vi "Load data.vi"(0 "File style in":u16(ring) items=["Sequential files", "Single database"], 1 "Fixed style":bool, 5 "Xcol in":i16, 7 "Ycol in":i16, 9 "Files in":path[](array[path]), 11 "Delim in":string) -> (4 "File style out":u16(ring) items=["Sequential files", "Single database"], 6 "Xcol out":i16, 8 "Ycol out":i16, 10 "Files out":path[](array[path]), 15 "Delim out":string)   [LabVIEW 2014]
panel:
  out "Delim":string
  in  "Ycol":i16=1
  in  "Xcol":i16
  out "Files":path[](array[path])
  in  "Process Stop Button":bool
  in  "File style":u16(ring) items=["Sequential files", "Single database"]
  in  "File delimit":u16(ring) items=["Tab", "Comma"]
  in  "Open Button":bool
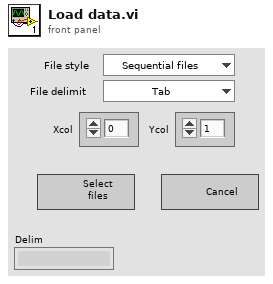
[diagram p1: front panel]
types:
  T1 = enum8{"Enabled", "Disabled", "Disabled and Grayed Out"}
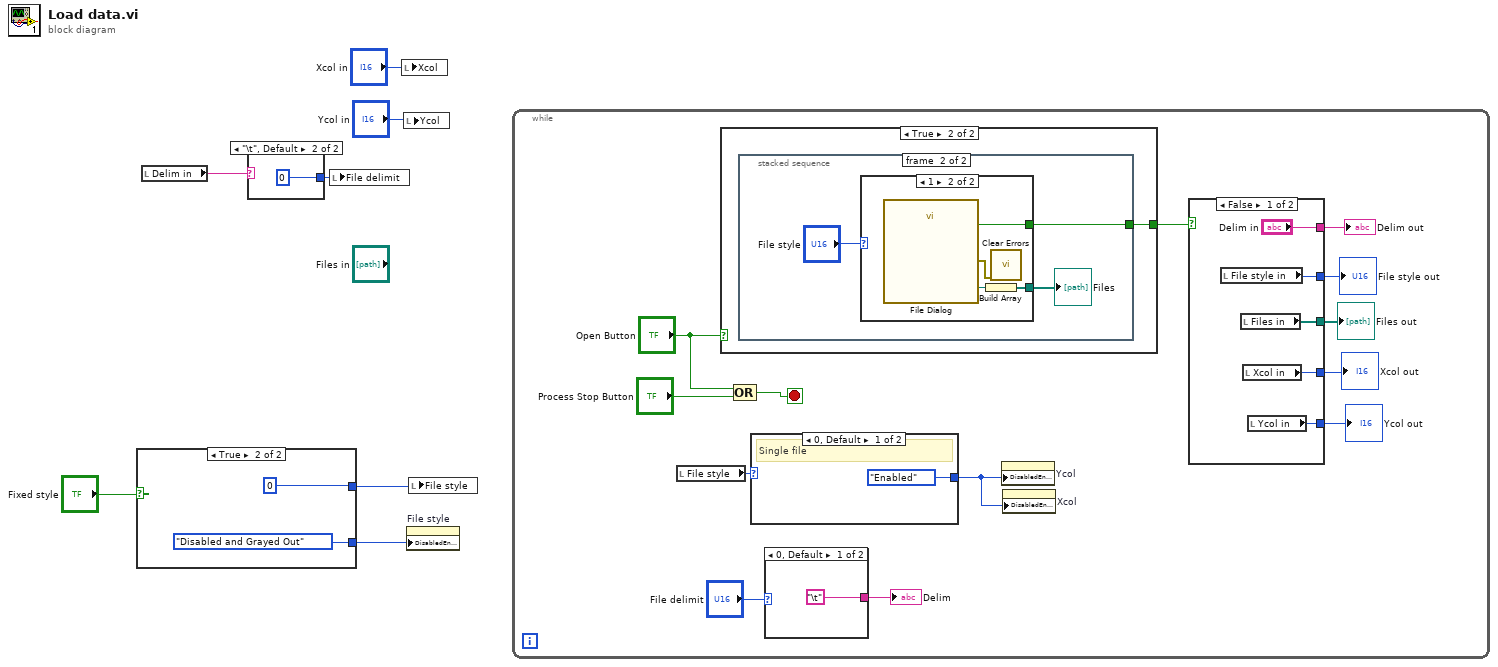
[diagram p0: block diagram]
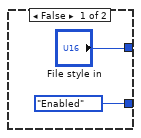
[diagram p2: hidden frame]
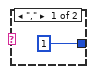
[diagram p3: hidden frame]
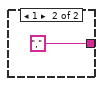
[diagram p4: hidden frame]
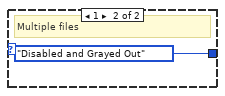
[diagram p5: hidden frame]
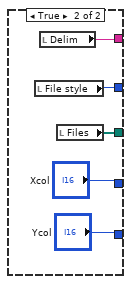
[diagram p6: hidden frame]
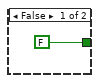
[diagram p7: hidden frame]
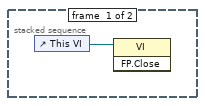
[diagram p8: hidden frame]
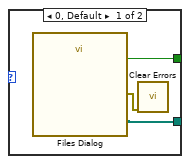
[diagram p9: hidden frame]
diagram:
  n1 = case shown="True" "Fixed style" {
    tunnel: ["File style in" 0] -> w2
    tunnel: [T1."Enabled" ("Disabled") T1."Disabled and Grayed Out" ("Disabled")] -> w1
    frame False {
    }
    frame True {
    }
  }
  n2 = local read "Delim in"() -> (w5:string)
  n3 = case shown="\"\\t\", Default" w5 {
    tunnel: [1 0] -> w4
    frame "," {
    }
    frame "\t", Default {
    }
  }
  n4 = local write "File delimit"(w4) -> ()
  n5 = local write "Xcol"("Xcol in") -> ()
  n6 = local write "Ycol"("Ycol in") -> ()
  n7 = property on="File style" class="Ring (strict)"("DisabledEnum"=w1) -> ()  [unwired: 2 in, 2 out]
  n8 = local write "File style"(w2) -> ()
  n9 = while {
    stop <- w21 stop-if-true
    n10 = local read "File style"() -> (w20:u16)
    n11 = case shown="True" "Open Button" {
      tunnel: [FALSE w42] -> w24
      frame False {
      }
      frame True {
        n12 = stacked-sequence {
          tunnel: [_ w44] -> w42
          frame #0 {
            n13 = control-ref of="This VI"() -> (w43:refnum<vi>)
            n14 = invoke class="VI" method="FP.Close"(reference=w43) -> ()  [unwired: 2 in, 3 out]
          }
          frame #1 {
            n15 = case shown="1" "File style" {
              tunnel: [w49 w53] -> w46
              tunnel: [w47 w50] -> w44
              frame 0, Default {
                n16 = call "Files Dialog"() -> ("selected paths"=w49:path[], "exists"=w47:bool, "error out"=w48:errorcluster)  [unwired: 12 in, 1 out]
                n17 = call <vilib>:"Clear Errors.vi"("error in (no error)"=w48) -> ()  [unwired: 5 in, 2 out]
              }
              frame 1 {
                n18 = call "File Dialog"() -> ("selected path"=w52:path, "exists"=w50:bool, "error out"=w51:errorcluster)  [unwired: 12 in, 1 out]
                n19 = Build Array(w52) -> (w53:path[])
                n20 = call <vilib>:"Clear Errors.vi"("error in (no error)"=w51) -> ()  [unwired: 5 in, 2 out]
              }
            }
            "Files" <- w46
          }
        }
      }
    }
    n21 = Compound Arithmetic op=OR("Open Button", "Process Stop Button") -> (w21:bool)
    n22 = case shown="0, Default" w20 {
      tunnel: [T1."Enabled" ("Disabled") T1."Disabled and Grayed Out" ("Disabled")] -> w19
      frame 0, Default {
        # "Single file"
      }
      frame 1 {
        # "Multiple files"
      }
    }
    n23 = case shown="0, Default" "File delimit" {
      tunnel: ["\t" ","] -> w17
      frame 0, Default {
      }
      frame 1 {
      }
    }
    "Delim" <- w17
    n24 = property on="Ycol" class="DigNum (strict)"("DisabledEnum"=w19) -> ()  [unwired: 2 in, 2 out]
    n25 = property on="Xcol" class="DigNum (strict)"("DisabledEnum"=w19) -> ()  [unwired: 2 in, 2 out]
    n26 = case shown="False" w24 {
      tunnel: [w34 w40] -> w26
      tunnel: [w35 w39] -> w25
      tunnel: ["Delim in" w38] -> w16
      tunnel: [w32 "Xcol"] -> w15
      tunnel: [w31 "Ycol"] -> w14
      frame False {
        n27 = local read "File style in"() -> (w35:u16)
        n28 = local read "Files in"() -> (w34:path[])
        n29 = local read "Xcol in"() -> (w32:i16)
        n30 = local read "Ycol in"() -> (w31:i16)
      }
      frame True {
        n31 = local read "File style"() -> (w39:u16)
        n32 = local read "Delim"() -> (w38:string)
        n33 = local read "Files"() -> (w40:path[])
      }
    }
    "File style out" <- w25
    "Files out" <- w26
    "Delim out" <- w16
    "Xcol out" <- w15
    "Ycol out" <- w14
  }
